vi "ma_FFT Spectrum no State (CDB).vi"(0 "time signal":waveform(cdb), 1 "restart averaging (F)":bool, 2 "mag-phase":bool, 5 "window":T3=1 items=["Rectangle"=0, "Hanning"=1, "Hamming"=2, "Blackman-Harris"=3, "Exact Blackman"=4, "Blackman"=5, "Flat Top"=6, "4 Term B-Harris "=7, "7 Term B-Harris"=8, "Low Sidelobe"=9, "Blackman Nuttall"=11, "Triangle"=30, "Bartlett-Hanning"=31, "Bohman"=32, "Parzen"=33, "Welch"=34, "Kaiser"=60, "Dolph-Chebyshev"=61, "Gaussian"=62], 7 "averaging parameters":T5={"averaging mode"=enum."No averaging", "weighting mode"=enum."Exponential", "number of averages"=10} {"number of averages" min=1}, 9 "view":T2, 11 "error in":errorcluster, 12 "state info":T4 {"real spectrum" format="%0.2f"; "averages completed" format="%0.2f"; "df" format="%0.2f"; "complex spectrum" format="%0.2f"; "spectrum parameters"."window" items=["Rectangle"=0, "Hanning"=1, "Hamming"=2, "Blackman-Harris"=3, "Exact Blackman"=4, "Blackman"=5, "Flat Top"=6, "4 Term B-Harris "=7, "7 Term B-Harris"=8, "Low Sidelobe"=9, "Blackman Nuttall"=11, "Triangle"=30, "Bartlett-Hanning"=31, "Bohman"=32, "Parzen"=33, "Welch"=34, "Kaiser"=60, "Dolph-Chebyshev"=61, "Gaussian"=62]; "dt" format="%0.2f"; "timestamp" format="%0.2f"; "dt history" format="%0.2f"; "t0 history" format="%0.2f"}, 13 "window parameter":dbl=nan) -> (3 "averaging done":bool, 4 "real or mag":cluster{"f0":dbl, "df":dbl, "real or mag":dbl[]} {"f0" format="%0.2p"; "df" format="%0.2p"; "real or mag" format="%0.2p"}, 6 "imag or phase":T1 {"f0" format="%0.2p"; "df" format="%0.2p"; "imag or phase" format="%0.2p"}, 10 "averages completed":dbl format="%0.2f", 14 "state info":T4 {"real spectrum" format="%0.2f"; "averages completed" format="%0.2f"; "df" format="%0.2f"; "complex spectrum" format="%0.2f"; "spectrum parameters"."window" items=["Rectangle"=0, "Hanning"=1, "Hamming"=2, "Blackman-Harris"=3, "Exact Blackman"=4, "Blackman"=5, "Flat Top"=6, "4 Term B-Harris "=7, "7 Term B-Harris"=8, "Low Sidelobe"=9, "Blackman Nuttall"=11, "Triangle"=30, "Bartlett-Hanning"=31, "Bohman"=32, "Parzen"=33, "Welch"=34, "Kaiser"=60, "Dolph-Chebyshev"=61, "Gaussian"=62]; "dt" format="%0.2f"; "timestamp" format="%0.2f"; "dt history" format="%0.2f"; "t0 history" format="%0.2f"}, 15 "error out":errorcluster)   [LabVIEW 2020, in "NI_MAPro.lvlib"]
doc: "Computes the averaged auto power spectrum of the input signal. Each time waveform corresponds to a single FFT block and has to be passed individually to this VI. Averaging parameters specifies how the averaging is performed. This includes the averaging mode (No averaging, vector averaging, RMS averaging, or peak hold), the weighting mode (linear or exponential), and the number of averages. Averages completed returns the number of averages completed so far."
uses:
  NI_MAPro.lvlib
  windowTd.ctl
  NI_MABase.lvlib
  NI_AALPro.lvlib
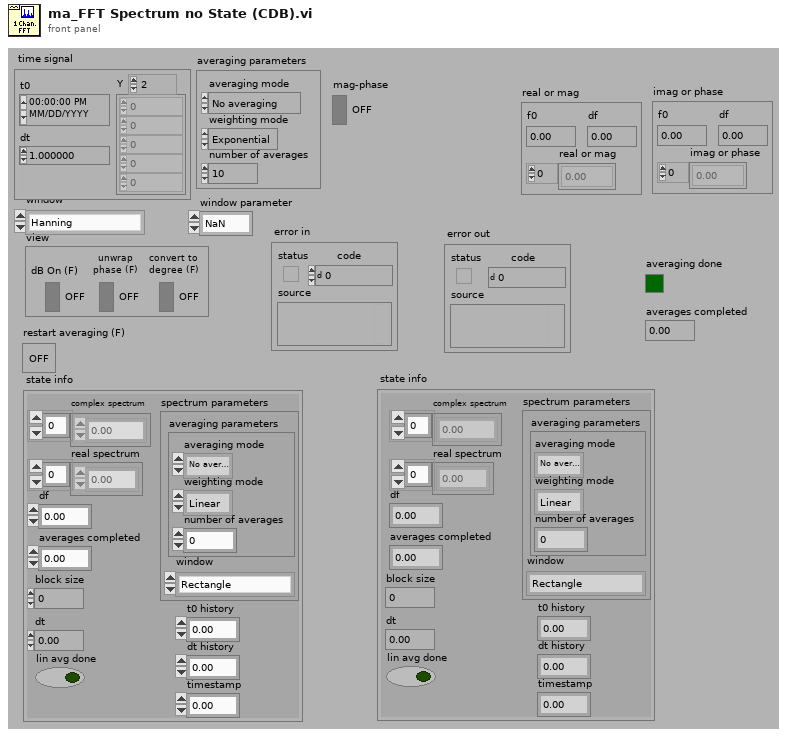
[diagram p1: front panel]
types:
  T1 = cluster{"f0":dbl, "df":dbl, "imag or phase":dbl[]}
  T2 = cluster{"dB On (F)":bool, "unwrap phase (F)":bool, "convert to degree (F)":bool}
  T3 = typedef "NI_AALPro.lvlib/windowTd.ctl" = u32
  T4 = cluster{"block size":i32, "dt":dbl, "spectrum parameters":cluster{"averaging parameters":cluster{"averaging mode":enum16{"No averaging", "Vector averaging", "RMS averaging", "Peak hold"}, "weighting mode":enum16{"Linear", "Exponential"}, "number of averages":u32}, "window":T3}, "df":dbl, "averages completed":dbl, "complex spectrum":cdb[], "real spectrum":dbl[], "t0 history":dbl, "dt history":dbl, "timestamp":dbl, "lin avg done":bool}
  T5 = cluster{"averaging mode":enum16{"No averaging", "Vector averaging", "RMS averaging", "Peak hold"}, "weighting mode":enum16{"Linear", "Exponential"}, "number of averages":u32}
  T6 = enum16{"FFT spectrum", "Power spectrum", "Cross spectrum", "Frequency response"}
  T7 = enum16{"No averaging", "Vector averaging", "RMS averaging", "Peak hold"}
  T8 = cluster{"f0":dbl, "df":dbl, "spectrum in dB":dbl[]}
  T9 = cluster{"f0":dbl, "df":dbl, "scaled phase":dbl[]}
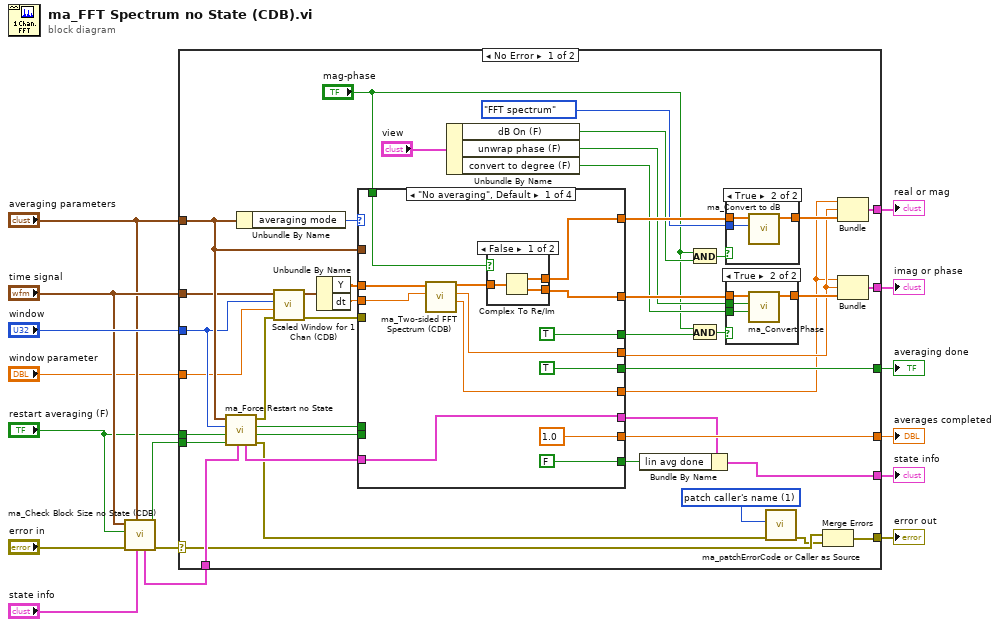
[diagram p0: block diagram]
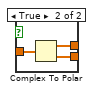
[diagram p4: hidden frame]
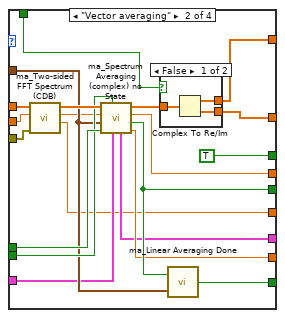
[diagram p5: hidden frame]
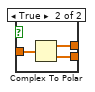
[diagram p6: hidden frame]
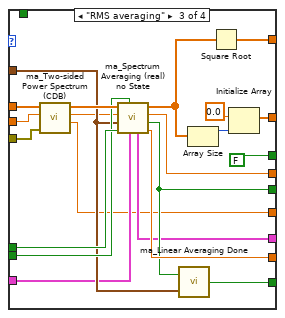
[diagram p7: hidden frame]
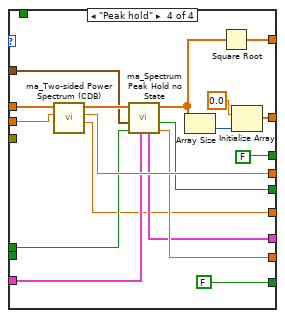
[diagram p8: hidden frame]
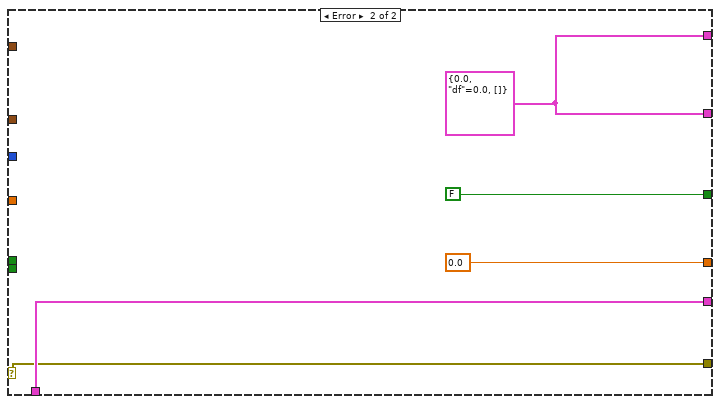
[diagram p9: hidden frame]
diagram:
  n1 = call "ma_Check Block Size no State (CDB).vi"("state info"="state info", "averaging parameters"="averaging parameters", "error in"="error in", "restart averaging (F)"="restart averaging (F)", "time signal"="time signal") -> ("error out"=w10:errorcluster, "force restart averaging"=w3:bool, "state info"=w6:T4)  [unwired: 1 in, 3 out]
  n2 = case shown="No Error" w10 {
    selector: w10 -> [w19 w153]
    tunnel: "averaging parameters" -> [w59 _]
    tunnel: [w58 0.0] -> w16
    tunnel: "window" -> [w57 _]
    tunnel: [w56 FALSE ("averaging done")] -> w14
    tunnel: "time signal" -> [w55 _]
    tunnel: "restart averaging (F)" -> [w54 _]
    tunnel: [w20 w153] -> w12
    tunnel: [w29 w154] -> w8
    tunnel: w6 -> [w42 w155]
    tunnel: [w52 w155] -> w5
    tunnel: [w30 w154] -> w4
    tunnel: w3 -> [w24 _]
    tunnel: "window parameter" -> [w21 _]
    frame No Error {
      w23 = u16 1 items=["patch error code", "patch caller's name"] ("operation")
      n3 = call "ma_Force Restart no State.vi"("state info"=w42, "force restart averaging in"=w24, "restart averaging (F)"=w54, "window"=w57, "averaging parameters"=w59) -> ("error out"=w18:errorcluster, "retrieve last spectrum"=w44:bool, "force restart averaging"=w45:bool, "skip processing"=w46:errorcluster, "state info"=w43:T4)  [unwired: 1 in, 1 out]
      n4 = Unbundle By Name(w59) -> ("averaging mode"=w51:T7)
      n5 = call "Scaled Window for 1 Chan (CDB).vi"("error in (no error)"=w46, "window parameter"=w21, "window"=w57, "signal in"=w55) -> ("error out"=w50:errorcluster, "signal out"=w47:waveform(cdb))  [unwired: 5 in, 1 out]
      n6 = Unbundle By Name(w47) -> ("Y"=w48:cdb[], "dt"=w49:dbl)
      n7 = case shown="\"No averaging\", Default" w51 {
        tunnel: w48 -> [w77 w105 w133 w152]
        tunnel: [w74 w92 w126 w150] -> w31
        tunnel: [w73 w90 w120 w141] -> w37
        tunnel: w59 -> [_ w99 w127 w144]
        tunnel: w45 -> [_ w107 w134 w148]
        tunnel: [1.0 ("averages completed") w96 w124 w147] -> w58
        tunnel: w49 -> [w76 w104 w132 w151]
        tunnel: [TRUE ("averaging done") w97 w123 w145] -> w56
        tunnel: [FALSE w102 w130 FALSE] -> w53
        tunnel: w50 -> [_ w101 w129 _]
        tunnel: w44 -> [_ w100 w128 _]
        tunnel: w43 -> [w78 w95 w122 w143]
        tunnel: [w78 w94 w121 w142] -> w41
        tunnel: [w72 w91 w116 w137] -> w36
        tunnel: [TRUE ("averaging done") TRUE FALSE FALSE] -> w32
        tunnel: "mag-phase" -> [w70 w89 _ _]
        tunnel: [w69 w88 w114 w135] -> w22
        frame "No averaging", Default {
          n8 = call "ma_Two-sided FFT Spectrum (CDB).vi"("dt"=w76, "signal (V)"=w77) -> ("f0"=w69:dbl, "df"=w74:dbl, "FFT spectrum (Vrms)"=w71:cdb[])  [unwired: 1 in, 6 out]
          n9 = case shown="False" w70 {
            tunnel: w71 -> [w84 w87]
            tunnel: [w83 w86] -> w73
            tunnel: [w82 w85] -> w72
            frame False {
              n10 = Complex To Re/Im(x + iy=w84) -> (x=w83:dbl[], y=w82:dbl[])
            }
            frame True {
              n11 = Complex To Polar(r * e^(i*theta)=w87) -> (r=w86:dbl[], theta=w85:dbl[])
            }
          }
        }
        frame "Vector averaging" {
          n12 = call "ma_Two-sided FFT Spectrum (CDB).vi"("error in"=w101, "dt"=w104, "signal (V)"=w105) -> ("f0"=w88:dbl, "df"=w98:dbl, "FFT spectrum (Vrms)"=w103:cdb[])  [unwired: 6 out]
          n13 = call "ma_Spectrum Averaging (complex) no State.vi"("state info"=w95, "retrieve last spectrum (F)"=w100, "restart averaging (F)"=w107, "averaging parameters"=w99, "df"=w98, "complex spectrum"=w103) -> ("averages completed"=w96:dbl, "averaging done"=w97:bool, "df"=w92:dbl, "averaged complex spectrum"=w106:cdb[], "state info"=w94:T4)  [unwired: 1 out]
          n14 = case shown="False" w89 {
            tunnel: w106 -> [w110 w113]
            tunnel: [w109 w112] -> w90
            tunnel: [w108 w111] -> w91
            frame False {
              n15 = Complex To Re/Im(x + iy=w110) -> (x=w109:dbl[], y=w108:dbl[])
            }
            frame True {
              n16 = Complex To Polar(r * e^(i*theta)=w113) -> (r=w112:dbl[], theta=w111:dbl[])
            }
          }
          n17 = call "ma_Linear Averaging Done.vi"("averaging parameters"=w99, "averaging done"=w97) -> ("linear averaging done"=w102:bool)
        }
        frame "RMS averaging" {
          n18 = call "ma_Two-sided Power Spectrum (CDB).vi"("error in"=w129, "dt"=w132, "signal (V)"=w133) -> ("f0"=w114:dbl, "df"=w125:dbl, "power spectrum (V^2 rms)"=w131:dbl[])  [unwired: 6 out]
          n19 = call "ma_Spectrum Averaging (real) no State.vi"("state info"=w122, "retrieve last spectrum (F)"=w128, "restart averaging (F)"=w134, "averaging parameters"=w127, "df"=w125, "real spectrum"=w131) -> ("averages completed"=w124:dbl, "averaging done"=w123:bool, "df"=w126:dbl, "averaged real spectrum"=w117:dbl[], "state info"=w121:T4)  [unwired: 1 out]
          n20 = call "ma_Linear Averaging Done.vi"("averaging parameters"=w127, "averaging done"=w123) -> ("linear averaging done"=w130:bool)
          n21 = Array Size(array=w117) -> (size(s)=w118:i32)
          n22 = Square Root(x=w117) -> (sqrt(x)=w120:dbl[])
          n23 = Initialize Array(0.0, w118) -> (w116:dbl[])
        }
        frame "Peak hold" {
          n24 = call "ma_Two-sided Power Spectrum (CDB).vi"("dt"=w151, "signal (V)"=w152) -> ("f0"=w135:dbl, "df"=w150:dbl, "power spectrum (V^2 rms)"=w149:dbl[])  [unwired: 1 in, 6 out]
          n25 = call "ma_Spectrum Peak Hold no State.vi"("state info"=w143, "restart averaging (F)"=w148, "averaging parameters"=w144, "real spectrum"=w149) -> ("averages completed"=w147:dbl, "averaging done"=w145:bool, "peak spectrum"=w138:dbl[], "state info"=w142:T4)  [unwired: 4 out]
          n26 = Array Size(array=w138) -> (size(s)=w139:i32)
          n27 = Square Root(x=w138) -> (sqrt(x)=w141:dbl[])
          n28 = Initialize Array(0.0, w139) -> (w137:dbl[])
        }
      }
      n29 = Unbundle By Name("view") -> ("dB On (F)"=w34:bool, "unwrap phase (F)"=w28:bool, "convert to degree (F)"=w27:bool)
      n30 = Bundle By Name(cluster=w41, "lin avg done"=w53) -> (w52:T4)
      n31 = And(x="mag-phase", y=w34) -> (x .and. y?=w35:bool)
      n32 = And(x="mag-phase", y=w32) -> (x .and. y?=w33:bool)
      n33 = case shown="True" w35 {
        tunnel: [w60 w62] -> w39
        tunnel: w37 -> [w60 w63]
        tunnel: T6."FFT spectrum" ("spectrum type") -> [_ w61]
        frame False {
        }
        frame True {
          n34 = call "ma_Convert to dB.vi"("spectrum type"=w61, "spectrum"=w63) -> ("spectrum in dB"=w62:dbl[])  [unwired: 9 out]
        }
      }
      n35 = case shown="True" w33 {
        tunnel: [w64 w65] -> w38
        tunnel: w36 -> [w64 w68]
        tunnel: w28 -> [_ w67]
        tunnel: w27 -> [_ w66]
        frame False {
        }
        frame True {
          n36 = call "ma_Convert Phase.vi"("convert to degree (F)"=w66, "unwrap phase (F)"=w67, "phase (radian)"=w68) -> ("scaled phase"=w65:dbl[])  [unwired: 3 in, 5 out]
        }
      }
      n37 = call "ma_patchErrorCode or Caller as Source.vi"("error in (no error)"=w18, "operation"=w23) -> ("error out"=w17:errorcluster)  [unwired: 2 in, 7 out]
      n38 = Merge Errors(w19, w17) -> (w20:errorcluster)
      n39 = Bundle("f0"=w22, "df"=w31, "spectrum in dB"=w39) -> (w29:T8)  [unwired: 1 out]
      n40 = Bundle("f0"=w22, "df"=w31, "scaled phase"=w38) -> (w30:T9)  [unwired: 1 out]
    }
    frame Error {
      w154 = cluster{dbl, "df":dbl, dbl[]} {0.0, "df"=0.0, []}
    }
  }
  "averages completed" <- w16
  "error out" <- w12
  "averaging done" <- w14
  "real or mag" <- w8
  "state info" <- w5
  "imag or phase" <- w4
